vi "top_rx.vi"(0 "Queues":T2, 1 "# of Receive Iterations":i32=1, 5 "HW parameters":T4={"Device IP Address"="192.168.11.6", "Active Antenna"="RX1", "Carrier Frequency (Hz)"=915000000.0, "Gain (dB)"=10.0, "Trigger Level"=0.01, "Bandwidth (Hz)"=40000000.0, "Reference Position (%)"=10.0, "Capture Time (s)"=0.0014, "Simulate"=FALSE} {"Capture Time (s)" format="%.2p"; "Bandwidth (Hz)" format="%.2p"; "Trigger Level" format="%#.3p"; "Gain (dB)" format="%.2f"; "Carrier Frequency (Hz)" format="%.2p"}, 7 "modulation parameters":T5={"modulation type"="QPSK", "pulse shaping parameters"={"modulation type"=enum."PSK", "pulse shaping filter"=enum."Raised Cosine", "filter parameter"=0.5, "filter length (symbols)"=8}, "control information\nfor packet header/tail"={"Training Sequence (derived)"=[0.7071067811865475+0.7071067811865475i, 0.7071067811865475+0.7071067811865475i, 0.7071067811865475+0.7071067811865475i, -0.7071067811865475-0.7071067811865475i, -0.7071067811865475-0.7071067811865475i, -0.7071067811865475-0.7071067811865475i, 0.7071067811865475+0.7071067811865475i, -0.7071067811865475-0.7071067811865475i, -0.7071067811865475-0.7071067811865475i, 0.7071067811865475+0.7071067811865475i, -0.7071067811865475-0.7071067811865475i, 0.7071067811865475+0.7071067811865475i, 0.7071067811865475+0.7071067811865475i, 0.7071067811865475+0.7071067811865475i, -0.7071067811865475-0.7071067811865475i, -0.7071067811865475-0.7071067811865475i, -0.7071067811865475-0.7071067811865475i, 0.7071067811865475+0.7071067811865475i, -0.7071067811865475-0.7071067811865475i, -0.7071067811865475-0.7071067811865475i, 0.7071067811865475+0.7071067811865475i, -0.7071067811865475-0.7071067811865475i, 0.7071067811865475+0.7071067811865475i, 0.7071067811865475+0.7071067811865475i, 0.7071067811865475+0.7071067811865475i, -0.7071067811865475-0.7071067811865475i, -0.7071067811865475-0.7071067811865475i, -0.7071067811865475-0.7071067811865475i, 0.7071067811865475+0.7071067811865475i, -0.7071067811865475-0.7071067811865475i, -0.7071067811865475-0.7071067811865475i, 0.7071067811865475+0.7071067811865475i, -0.7071067811865475-0.7071067811865475i, 0.7071067811865475+0.7071067811865475i, 0.7071067811865475+0.7071067811865475i, 0.7071067811865475+0.7071067811865475i, -0.7071067811865475-0.7071067811865475i, -0.7071067811865475-0.7071067811865475i, -0.7071067811865475-0.7071067811865475i, 0.7071067811865475+0.7071067811865475i, -0.7071067811865475-0.7071067811865475i, -0.7071067811865475-0.7071067811865475i, 0.7071067811865475+0.7071067811865475i, -0.7071067811865475-0.7071067811865475i], "Zero Pad Length"=8}, "RX oversample factor"=10, "channel estimation/equalizer\nparameters"={"channel estimate length"=2, "equalizer length"=1, "equalizer delay"=-1, "Equalization Method"="Direct"}, "synchronization options"={"Symbol Timing Recovery Method"="Max Energy", "Synchronization Method"="Timing Estimation", "Correct Frequency Offset"=FALSE, "fixed offset"=0, "Frame Detection Method"="Sliding Correlator"}, "number of data \nsymbols (derived)"=250, "RX Sample Rate"=1000000.0} {"RX Sample Rate" items=["25M"=25000000.0, "20M"=20000000.0, "16.6667M"=16666666.666667, "14.2857M"=14285714.285714, "12.5M"=12500000.0, "11.1111M"=11111111.111111, "10M"=10000000.0, "9.09091M"=9090909.090909, "8.33333M"=8333333.333333, "7.69231M"=7692307.692308, "7.14286M"=7142857.142857, "6.66667M"=6666666.666667, "6.25M"=6250000.0, "5.88235M"=5882352.941176, "5.55556M"=5555555.555556, "5.26316M"=5263157.894737, "5M"=5000000.0, "4.7619M"=4761904.761905, "4.54545M"=4545454.545455, "4.34783M"=4347826.086957, "4.16667M"=4166666.666667, "4M"=4000000.0, "3.84615M"=3846153.846154, "3.7037M"=3703703.703704, "3.57143M"=3571428.571429, "3.44828M"=3448275.862069, "3.33333M"=3333333.333333, "3.22581M"=3225806.451613, "3.125M"=3125000.0, "3.0303M"=3030303.030303, "2.94118M"=2941176.470588, "2.85714M"=2857142.857143, "2.77778M"=2777777.777778, "2.7027M"=2702702.702703, "2.63158M"=2631578.947368, "2.5641M"=2564102.564103, "2.5M"=2500000.0, "2.43902M"=2439024.390244, "2.38095M"=2380952.380952, "2.32558M"=2325581.395349, "2.27273M"=2272727.272727, "2.22222M"=2222222.222222, "2.17391M"=2173913.043478, "2.12766M"=2127659.574468, "2.08333M"=2083333.333333, "2.04082M"=2040816.326531, "2M"=2000000.0, "1.96078M"=1960784.313725, "1.92308M"=1923076.923077, "1.88679M"=1886792.45283, "1.85185M"=1851851.851852, "1.81818M"=1818181.818182, "1.78571M"=1785714.285714, "1.75439M"=1754385.964912, "1.72414M"=1724137.931034, "1.69492M"=1694915.254237, "1.66667M"=1666666.666667, "1.63934M"=1639344.262295, "1.6129M"=1612903.225806, "1.5873M"=1587301.587302, "1.5625M"=1562500.0, "1.53846M"=1538461.538462, "1.51515M"=1515151.515152, "1.49254M"=1492537.313433, "1.47059M"=1470588.235294, "1.44928M"=1449275.362319, "1.42857M"=1428571.428571, "1.40845M"=1408450.704225, "1.38889M"=1388888.888889, "1.36986M"=1369863.013699, "1.35135M"=1351351.351351, "1.33333M"=1333333.333333, "1.31579M"=1315789.473684, "1.2987M"=1298701.298701, "1.28205M"=1282051.282051, "1.26582M"=1265822.78481, "1.25M"=1250000.0, "1.23457M"=1234567.901235, "1.21951M"=1219512.195122, "1.20482M"=1204819.277108, "1.19048M"=1190476.190476, "1.17647M"=1176470.588235, "1.16279M"=1162790.697674, "1.14943M"=1149425.287356, "1.13636M"=1136363.636364, "1.1236M"=1123595.505618, "1.11111M"=1111111.111111, "1.0989M"=1098901.098901, "1.08696M"=1086956.521739, "1.07527M"=1075268.817204, "1.06383M"=1063829.787234, "1.05263M"=1052631.578947, "1.04167M"=1041666.666667, "1.03093M"=1030927.835052, "1.02041M"=1020408.163265, "1.0101M"=1010101.010101, "1M"=1000000.0, "990.099k"=990099.009901, "980.392k"=980392.156863, "970.874k"=970873.786408, "961.538k"=961538.461538, "952.381k"=952380.952381, "943.396k"=943396.226415, "934.579k"=934579.439252, "925.926k"=925925.925926, "917.431k"=917431.192661, "909.091k"=909090.909091, "900.901k"=900900.900901, "892.857k"=892857.142857, "884.956k"=884955.752212, "877.193k"=877192.982456, "869.565k"=869565.217391, "862.069k"=862068.965517, "854.701k"=854700.854701, "847.458k"=847457.627119, "840.336k"=840336.134454, "833.333k"=833333.333333, "826.446k"=826446.280992, "819.672k"=819672.131148, "813.008k"=813008.130081, "806.452k"=806451.612903, "800k"=800000.0, "793.651k"=793650.793651, "787.402k"=787401.574803, "781.25k"=781250.0, "769.231k"=769230.769231, "757.576k"=757575.757576, "746.269k"=746268.656716, "735.294k"=735294.117647, "724.638k"=724637.681159, "714.286k"=714285.714286, "704.225k"=704225.352113, "694.444k"=694444.444444, "684.932k"=684931.506849, "675.676k"=675675.675676, "666.667k"=666666.666667, "657.895k"=657894.736842, "649.351k"=649350.649351, "641.026k"=641025.641026, "632.911k"=632911.392405, "625k"=625000.0, "617.284k"=617283.950617, "609.756k"=609756.097561, "602.41k"=602409.638554, "595.238k"=595238.095238, "588.235k"=588235.294118, "581.395k"=581395.348837, "574.713k"=574712.643678, "568.182k"=568181.818182, "561.798k"=561797.752809, "555.556k"=555555.555556, "549.451k"=549450.549451, "543.478k"=543478.26087, "537.634k"=537634.408602, "531.915k"=531914.893617, "526.316k"=526315.789474, "520.833k"=520833.333333, "515.464k"=515463.917526, "510.204k"=510204.081633, "505.051k"=505050.505051, "500k"=500000.0, "495.05k"=495049.50495, "490.196k"=490196.078431, "485.437k"=485436.893204, "480.769k"=480769.230769, "476.19k"=476190.47619, "471.698k"=471698.113208, "467.29k"=467289.719626, "462.963k"=462962.962963, "458.716k"=458715.59633, "454.545k"=454545.454545, "450.45k"=450450.45045, "446.429k"=446428.571429, "442.478k"=442477.876106, "438.596k"=438596.491228, "434.783k"=434782.608696, "431.034k"=431034.482759, "427.35k"=427350.42735, "423.729k"=423728.813559, "420.168k"=420168.067227, "416.667k"=416666.666667, "413.223k"=413223.140496, "409.836k"=409836.065574, "406.504k"=406504.065041, "403.226k"=403225.806452, "400k"=400000.0, "396.825k"=396825.396825, "393.701k"=393700.787402, "390.625k"=390625.0, "384.615k"=384615.384615, "378.788k"=378787.878788, "373.134k"=373134.328358, "367.647k"=367647.058824, "362.319k"=362318.84058, "357.143k"=357142.857143, "352.113k"=352112.676056, "347.222k"=347222.222222, "342.466k"=342465.753425, "337.838k"=337837.837838, "333.333k"=333333.333333, "328.947k"=328947.368421, "324.675k"=324675.324675, "320.513k"=320512.820513, "316.456k"=316455.696203, "312.5k"=312500.0, "308.642k"=308641.975309, "304.878k"=304878.04878, "301.205k"=301204.819277, "297.619k"=297619.047619, "294.118k"=294117.647059, "290.698k"=290697.674419, "287.356k"=287356.321839, "284.091k"=284090.909091, "280.899k"=280898.876404, "277.778k"=277777.777778, "274.725k"=274725.274725, "271.739k"=271739.130435, "268.817k"=268817.204301, "265.957k"=265957.446809, "263.158k"=263157.894737, "260.417k"=260416.666667, "257.732k"=257731.958763, "255.102k"=255102.040816, "252.525k"=252525.252525, "250k"=250000.0, "247.525k"=247524.752475, "245.098k"=245098.039216, "242.718k"=242718.446602, "240.385k"=240384.615385, "238.095k"=238095.238095, "235.849k"=235849.056604, "233.645k"=233644.859813, "231.481k"=231481.481481, "229.358k"=229357.798165, "227.273k"=227272.727273, "225.225k"=225225.225225, "223.214k"=223214.285714, "221.239k"=221238.938053, "219.298k"=219298.245614, "217.391k"=217391.304348, "215.517k"=215517.241379, "213.675k"=213675.213675, "211.864k"=211864.40678, "210.084k"=210084.033613, "208.333k"=208333.333333, "206.612k"=206611.570248, "204.918k"=204918.032787, "203.252k"=203252.03252, "201.613k"=201612.903226, "200k"=200000.0, "198.413k"=198412.698413, "196.85k"=196850.393701, "195.312k"=195312.5]; "control information\nfor packet header/tail"."Training Sequence (derived)" format="%#_3p"}, 9 "Received IQ\nwaveform":cluster{"t0":dbl, "dt":dbl, "Y":cdb[]} {"Y" format="%.2g"; "dt" format="%.2g"; "t0" format="%.2g"}, 11 "error in":errorcluster) -> (2 "Measured channel impairements":T1, 3 "average \nbit-error rate":dbl, 4 "I Data":waveform(dbl)(graph)={"t0"=timestamp(-0.00019717187500001288 s since 1904-01-01), "dt"=5e-07, "Y"=[]}, 6 "Q Data":waveform(dbl)(graph)={"t0"=timestamp(-0.00019717187500001288 s since 1904-01-01), "dt"=5e-07, "Y"=[]}, 8 "Eye Diagram":cluster{"t0":dbl, "dt":dbl, "Y":dbl[]}[](graph), 10 "Received\n Constellation":cluster{dbl[], dbl[]}(graph), 13 "offset":i32, 14 "Power Delay Profile":waveform(dbl)(graph), 15 "error out":errorcluster)   [LabVIEW 2009]
doc: "This example shows how you can configure the NI PXI-5660 for IQ acquisition and analysis."
uses:
  control_type_defs.llb/rx_hw params.ctl
  control_type_defs.llb/rx_modulation params.ctl
  control_type_defs.llb/Queues.ctl
  <vilib>/Analysis/NI_AALBase.lvlib
  <vilib>/addons/Modulation/niAMT.lvlib
panel:
  in  "stop":bool
  out "symbol rate":dbl format="%#_6p"
  out "coerced gain (dB)":dbl format="%#_6f"
  out "coerced carrier frequency (Hz)":dbl format="%#_6p"
  out "coerced bandwidth":dbl
  out "bit-error rate":dbl
  out "overhead offset":i32
  out "key bit sequence":u8[](array[numeric])
  in  "Tab Control 2":T3(tab)
  in  "Tab Control":enum32{"HW parameters", "modulation parameters"}(tab)
  out "Packet Detected":bool
  # "( set delay to -1 for equalizer\n  to choose optimal delay )"
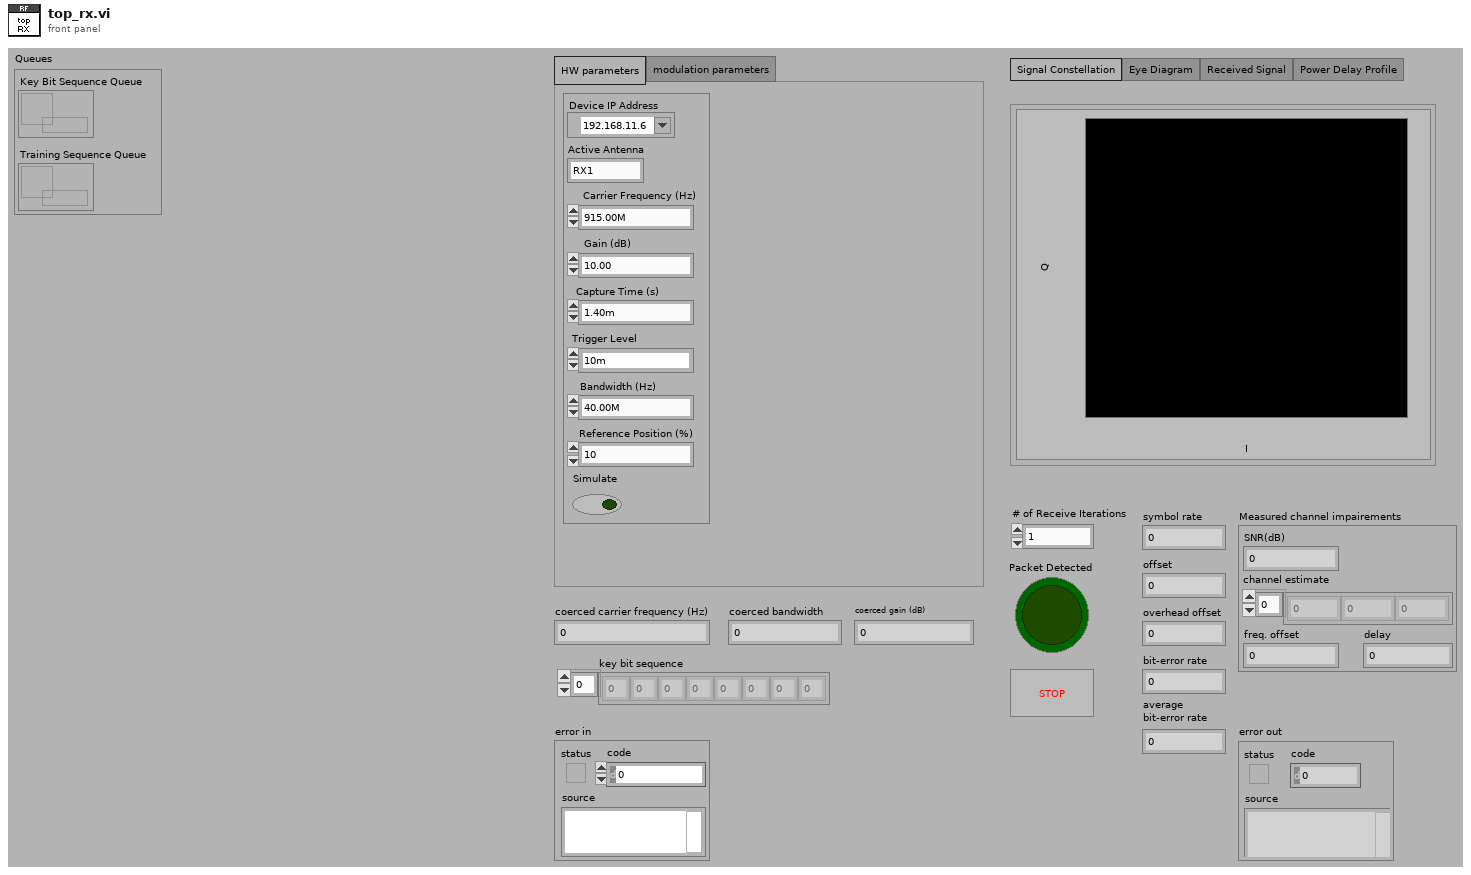
[diagram p1: front panel]
types:
  T1 = cluster{"SNR(dB)":dbl, "channel estimate":cdb[], "freq. offset":dbl, "delay":dbl}
  T2 = typedef "Queues.ctl" = cluster{"Key Bit Sequence Queue":refnum<queue>, "Training Sequence Queue":refnum<queue>}
  T3 = enum32{"Signal Constellation", "Eye Diagram", "Received Signal", "Power Delay Profile"}
  T4 = typedef "rx_hw params.ctl" = cluster{"Device IP Address":refnum<k15>, "Active Antenna":string, "Carrier Frequency (Hz)":dbl, "Gain (dB)":dbl, "Trigger Level":dbl, "Bandwidth (Hz)":dbl, "Reference Position (%)":dbl, "Capture Time (s)":dbl, "Simulate":bool}
  T5 = typedef "rx_modulation params.ctl" = cluster{"modulation type":string, "pulse shaping parameters":cluster{"modulation type":enum16{"FSK", "PSK", "QAM", "MSK", "PAM", "ASK"}, "pulse shaping filter":enum16{"none", "Raised Cosine", "Root Raised Cos", "Gaussian"}, "filter parameter":dbl, "filter length (symbols)":i32}, "control information\nfor packet header/tail":cluster{"Training Sequence (derived)":cdb[], "Zero Pad Length":i32}, "RX oversample factor":i32, "channel estimation/equalizer\nparameters":cluster{"channel estimate length":i32, "equalizer length":i32, "equalizer delay":i32, "Equalization Method":string}, "synchronization options":cluster{"Symbol Timing Recovery Method":string, "Synchronization Method":string, "Correct Frequency Offset":bool, "fixed offset":i32, "Frame Detection Method":string}, "number of data \nsymbols (derived)":i32, "RX Sample Rate":dbl}
  T6 = typedef "niAMT.lvlib/Complex Data Waveform.ctl" = cluster{"t0":dbl, "dt":dbl, "Y":cdb[]}
  T7 = cluster{"IQ Graph":cluster{dbl[], dbl[]}, "eye diagram":cluster{"t0":dbl, "dt":dbl, "Y":dbl[]}[], "Power Delay Profile":waveform(dbl)}
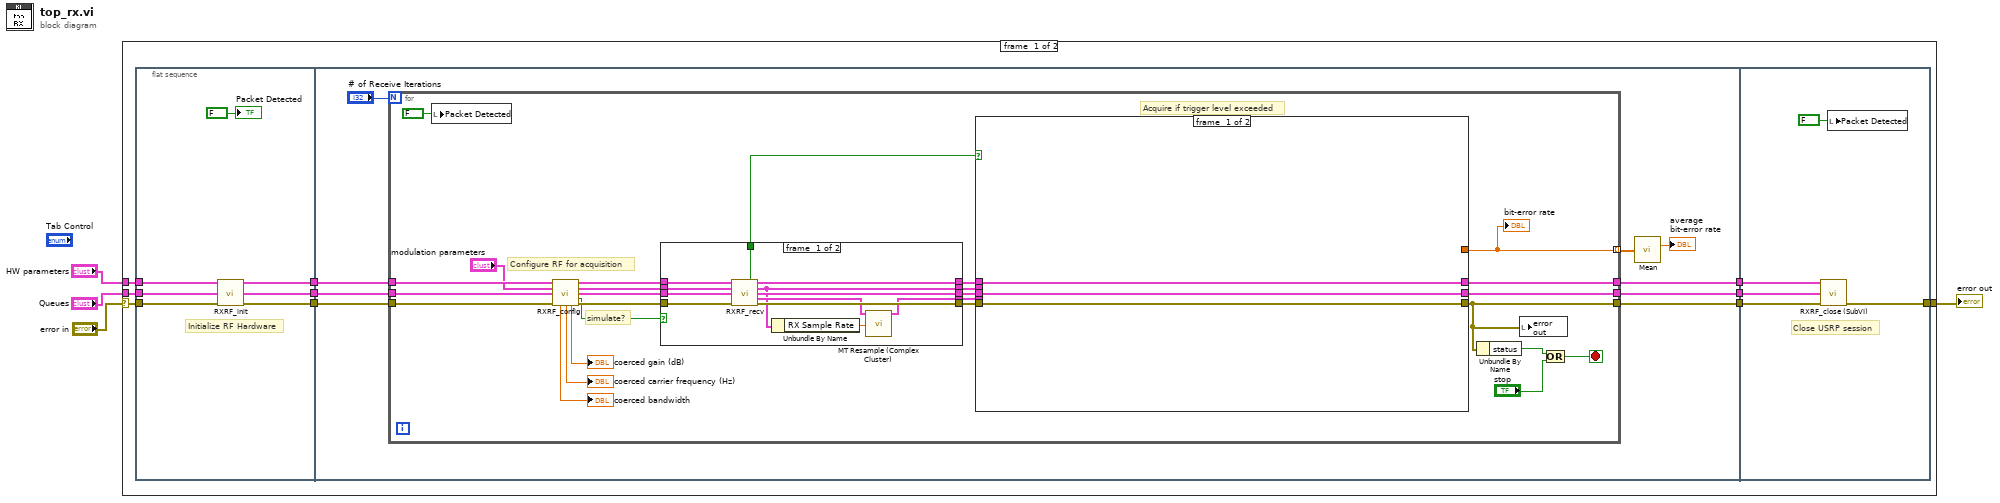
[diagram p0: block diagram]
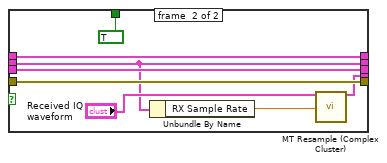
[diagram p2: hidden frame]
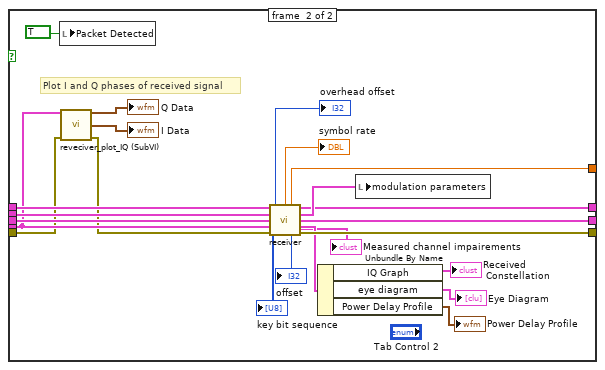
[diagram p3: hidden frame]
diagram:
  n1 = case shown="No Error" "error in" {
    selector: "error in" -> [w9 w108]
    tunnel: [w10 w108] -> w4
    tunnel: "HW parameters" -> [w8 _]
    tunnel: "Queues" -> [w7 _]
    frame #0 {
      n2 = flat-sequence {
        tunnel: [w19] -> w14
        tunnel: [w20] -> w13
        tunnel: w9 -> [w18]
        tunnel: w8 -> [w17]
        tunnel: w7 -> [w16]
        tunnel: [w15] -> w6
        tunnel: w14 -> [w28]
        tunnel: w13 -> [w27]
        tunnel: [w30] -> w12
        tunnel: [w29] -> w11
        tunnel: w6 -> [w26]
        tunnel: [w25] -> w5
        tunnel: w12 -> [w105]
        tunnel: w11 -> [w106]
        tunnel: [w104] -> w10
        tunnel: w5 -> [w103]
        frame #0 {
          # "Initialize RF Hardware"
          n3 = call "RXRF_init.vi"("HW parameters in"=w17, "Queues in"=w16, "error in (no error)"=w18) -> ("HW parameters out"=w20:T4, "Queues out"=w15:T2, "error out"=w19:errorcluster)  [unwired: 9 in, 1 out]
          "Packet Detected" <- FALSE ("Boolean")
        }
        frame #1 {
          n4 = for {
            N: "# of Receive Iterations" -> [_]
            tunnel: [w56] -> w30
            tunnel: [w34] -> w29
            tunnel: w28 -> [w55]
            tunnel: w27 -> [w54]
            tunnel: w26 -> [w53]
            tunnel: [w52] -> w25
            tunnel: [w38] -> w23 mode=indexing
            stop <- w33 stop-if-true
            # "simulate?"
            # "Acquire if trigger level exceeded"
            # "Configure RF for acquisition"
            n5 = local write "Packet Detected"(FALSE ("Packet Detected?")) -> ()
            n6 = call "RXRF_config.vi"("HW parameters in"=w54, "modulation parameters in"="modulation parameters", "Queues in"=w53, "error in (no error)"=w55) -> ("HW parameters out"=w47:T4, "modulation parameters out"=w46:T5, "Queues out"=w44:T2, "Simulate"=w39:bool, "coerced bandwidth"=→"coerced bandwidth":dbl, "coerced carrier frequency (Hz)"=→"coerced carrier frequency (Hz)":dbl, "coerced gain (dB)"=→"coerced gain (dB)":dbl, "error out"=w50:errorcluster)  [unwired: 4 in]
            n7 = case shown="False" w39 {
              tunnel: w50 -> [w68 w74]
              tunnel: [w57 w71] -> w41
              tunnel: [w67 w74] -> w40
              tunnel: [w66 w76] -> w49
              tunnel: [w65 TRUE ("Packet Detected")] -> w48
              tunnel: w47 -> [w64 w76]
              tunnel: w46 -> [w63 w70]
              tunnel: [w58 w70] -> w45
              tunnel: w44 -> [w62 w75]
              tunnel: [w61 w75] -> w43
              frame #0 {
                n8 = call "RXRF_recv.vi"("HW parameters in"=w64, "modulation parameters in"=w63, "Queues in"=w62, "error in (no error)"=w68) -> ("Packet Detected"=w65:bool, "HW parameters out"=w66:T4, "modulation parameters out"=w58:T5, "Queues out"=w61:T2, "Received IQ waveform"=w59:cluster{"t0":dbl, "dt":dbl, "Y":cdb[]}, "error out"=w67:errorcluster)  [unwired: 6 in]
                n9 = Unbundle By Name(w58) -> ("RX Sample Rate"=w60:dbl)
                n10 = call <vilib>:"MT Resample (Complex Cluster).vi"("input complex waveform"=w59, "desired sample rate (Hz)"=w60) -> ("output complex waveform"=w57:T6)  [unwired: 12 in, 1 out]
              }
              frame #1 {
                n11 = Unbundle By Name(w70) -> ("RX Sample Rate"=w69:dbl)
                n12 = call <vilib>:"MT Resample (Complex Cluster).vi"("input complex waveform"="Received IQ\nwaveform", "desired sample rate (Hz)"=w69) -> ("output complex waveform"=w71:T6)  [unwired: 12 in, 1 out]
              }
            }
            n13 = case shown="True" w48 {
              tunnel: w41 -> [_ w85]
              tunnel: [w77 w101] -> w34
              tunnel: w49 -> [w79 w97]
              tunnel: w45 -> [_ w96]
              tunnel: w43 -> [w78 w95]
              tunnel: [w78 w94] -> w52
              tunnel: [w79 w81] -> w56
              tunnel: w40 -> [w77 w84]
              tunnel: [_ w80] -> w38
              frame #0 {
              }
              frame #1 {
                # "Plot I and Q phases of received signal"
                n14 = local write "Packet Detected"(TRUE ("Packet Detected?")) -> ()
                n15 = call "reveciver_plot_IQ (SubVI).vi"("Received IQ\nwaveform"=w85, "error in"=w84) -> ("Q"=→"Q Data":waveform(dbl), "I"=→"I Data":waveform(dbl), "error out"=w83:errorcluster)  [unwired: 11 in]
                n16 = call "receiver.vi"("HW parameters in"=w97, "modulation parameters"=w96, "Queues in"=w95, "input complex waveform"=w85, "error in (no error)"=w83) -> ("overhead offset"=→"overhead offset":i32, "symbol rate"=→"symbol rate":dbl, "bit-error rate"=w80:dbl, "HW parameters out"=w81:T4, "modulation parameters out"=w100:T5, "Queues out"=w94:T2, "RX waveforms out"=w99:T7, "Measured channel impairements"=→"Measured channel impairements":T1, "key bit sequence"=→"key bit sequence":u8[], "offset"=→"offset":i32, "error out"=w101:errorcluster)
                n17 = Unbundle By Name(w99) -> ("IQ Graph"=→"Received\n Constellation":cluster{dbl[], dbl[]}, "eye diagram"=→"Eye Diagram":cluster{"t0":dbl, "dt":dbl, "Y":dbl[]}[], "Power Delay Profile"=→"Power Delay Profile":waveform(dbl))
                n18 = local write "modulation parameters"(w100) -> ()
              }
            }
            "bit-error rate" <- w38
            n19 = Unbundle By Name(w34) -> ("status"=w32:bool)
            n20 = local write "error out"(w34) -> ()
            n21 = Or(x=w32, y="stop") -> (x .or. y?=w33:bool)
          }
          n22 = call <vilib>:"Mean.vi"("X"=w23) -> ("mean"=→"average \nbit-error rate":dbl)  [unwired: 1 out]
        }
        frame #2 {
          # "Close USRP session"
          n23 = call "RXRF_close (SubVI).vi"("HW parameters in"=w105, "Queues in"=w103, "error in"=w106) -> ("error out"=w104:errorcluster)  [unwired: 12 in]
          n24 = local write "Packet Detected"(FALSE ("Packet Detected?")) -> ()
        }
      }
    }
    frame #1 {
    }
  }
  "error out" <- w4
